vi "GetData.vi"() -> (2 "data":string[][](array[string]))   [LabVIEW 2020]
uses:
  <vilib>/addons/database/Connection.llb/DB Tools Open Connec (Path).vi
  <vilib>/addons/database/_DB Variant To Data/Database Variant To Data.xnode
  <vilib>/addons/database/NI_Database_API.lvlib
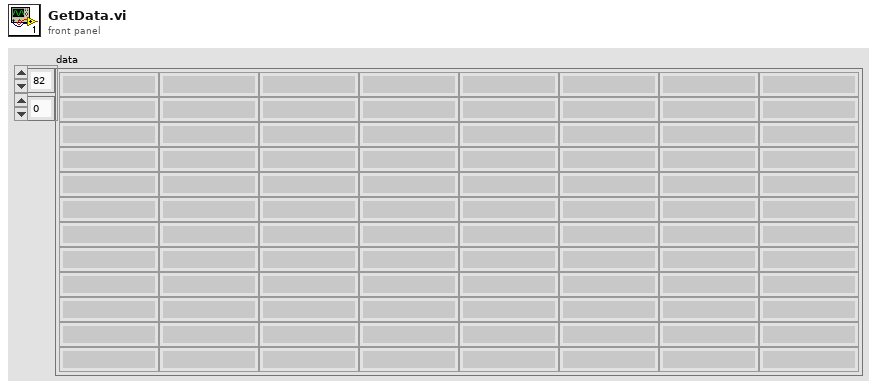
[diagram p1: front panel]
types:
  T1 = typedef "NI_Database_API.lvlib/Conn ObjectReference.ctl" = refnum<k1>
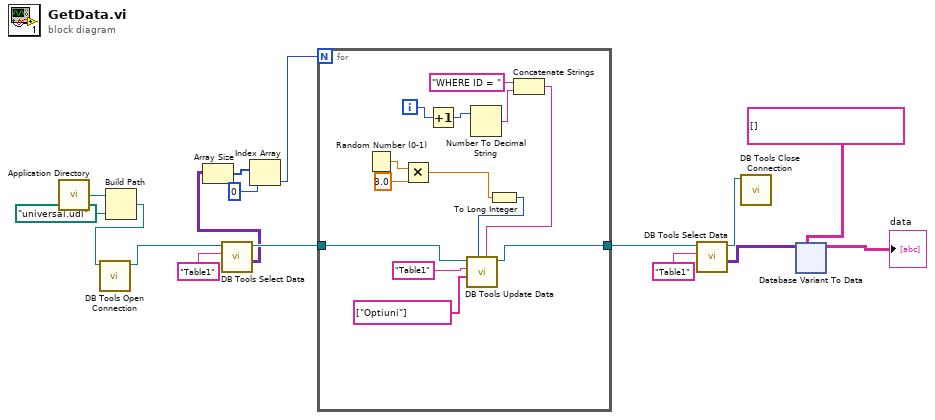
[diagram p0: block diagram]
diagram:
  n1 = call <vilib>:"Application Directory.vi"() -> ("Application Directory"=w15:path)
  n2 = Build Path(base path=w15, name or relative path=path "universal.udl") -> (appended path=w13:path)
  n3 = call-poly <vilib>:"DB Tools Open Connection.vi"("connection information"=w13) -> ("connection reference"=w6:T1)  [unwired: 7 in, 1 out]
  n4 = call <vilib>:"DB Tools Select Data.vi"("table"="Table1", "connection reference"=w6) -> ("data"=w4:variant[][], "connection reference out"=w5:T1)  [unwired: 4 in, 1 out]
  n5 = Array Size(array=w4) -> (size(s)=w3:i32[])
  n6 = Index Array(array=w3, index=0) -> (element=w1:i32)
  n7 = for {
    N: w1 -> [_]
    tunnel: w5 -> [w28]
    tunnel: [w27] -> w12
    i -> [w18]
    n8 = Random Number (0-1)() -> (number: 0 to 1=w25:dbl)
    n9 = Multiply(x=w25, y=3.0) -> (x*y=w23:dbl)
    n10 = Increment(x=w18) -> (x+1=w17:i32)
    n11 = Number To Decimal String(number=w17) -> (decimal integer string=w20:string)  [unwired: 1 in]
    n12 = To Long Integer(number=w23) -> (32bit integer=w22:i32)
    n13 = Concatenate Strings("WHERE ID = " ("string"), w20) -> (w19:string)
    n14 = call <vilib>:"DB Tools Update Data.vi"("condition"=w19, "data"=w22, "columns"=string[] ["Optiuni"], "table"="Table1", "connection reference"=w28) -> ("connection reference out"=w27:T1)  [unwired: 5 in, 1 out]
  }
  n15 = call <vilib>:"DB Tools Select Data.vi"("table"="Table1", "connection reference"=w12) -> ("data"=w10:variant[][], "connection reference out"=w11:T1)  [unwired: 4 in, 1 out]
  n16 = call <vilib>:"DB Tools Close Connection.vi"("connection reference"=w11) -> ()  [unwired: 6 in, 1 out]
  n17 = xnode "Database Variant To Data"("database variant"=w10, "type"=string[][] []) -> ("data"=→"data":string[][])  [unwired: 1 in, 1 out]
